vi "Start.vi"(5 "Autoshutdown? (T)":bool=TRUE, 7 "StartupParams":variant, 8 "error in (no error)":errorcluster, 11 "JQMHCore in":refnum<class "JQMHModule.lvclass">) -> (0 "error out":errorcluster, 3 "JQMHCore out":refnum<class "JQMHModule.lvclass">)   [LabVIEW 2024, in "JQMHModule.lvclass"]
uses:
  JQMHModule.lvclass
  JQMHModule.lvclass/JQMHModule.ctl
  JQMHStartup/JQMHStartup.lvclass
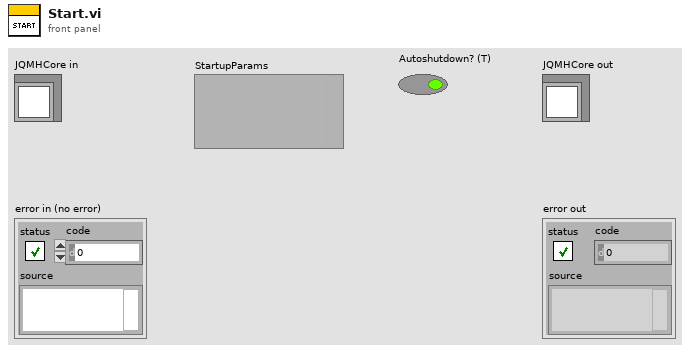
[diagram p1: front panel]
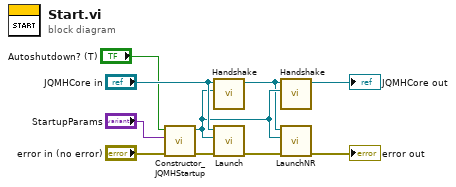
[diagram p0: block diagram]
diagram:
  n1 = call "Constructor_JQMHStartup.vi"("error in (no error)"="error in (no error)", "StartupParams"="StartupParams", "Autoshutdown? (T)"="Autoshutdown? (T)") -> ("error out"=w9:errorcluster, "JQMHStartup out"=w6:refnum<class "JQMHStartup.lvclass">)  [unwired: 7 in]
  n2 = call "Handshake.vi"("JQMHStartup in"=w6, "JQMHModule in"="JQMHCore in") -> ("JQMHModule out"=w5:refnum<class "JQMHModule.lvclass">)  [unwired: 8 in, 1 out]
  n3 = call "Launch.vi"("error in (no error)"=w9, "JQMHStartup"=w6, "JQMHCore in"="JQMHCore in") -> ("error out"=w7:errorcluster)  [unwired: 8 in]
  n4 = call "Handshake.vi"("JQMHStartup in"=w6, "JQMHModule in"=w5) -> ("JQMHModule out"=→"JQMHCore out":refnum<class "JQMHModule.lvclass">)  [unwired: 8 in, 1 out]
  n5 = call "LaunchNR.vi"("error in (no error)"=w7, "JQMHStartup"=w6, "JQMHCore in"=w5) -> ("error out"=→"error out":errorcluster)  [unwired: 8 in]
